vi "Receive Dashboard Packet.vi"(7 "connection ID":refnum<k16>) -> ()   [LabVIEW 2015]
uses:
  Common Code/Dashboard Communication/Dashboard Control Data.ctl
  Common Code/Shooter Presets.ctl
  Common Code/Shot Presets.ctl
  Common Code/Encoder Control.ctl
  Common Code/Drivetrain Settings.ctl
  Common Code/Vision Packet.ctl
  Common Code/Dashboard Drivetrain Command.ctl
  Common Code/Drivetrain Vision.ctl
  Robot Global Data.vi
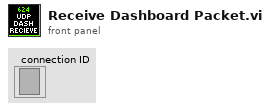
[diagram p1: front panel]
types:
  T1 = typedef "Dashboard Control Data.ctl" = cluster{"Auton Loops":dbl, "Shooter Presets":T2, "Encoder Control":T4, "Steer PID output":cluster{"output high":dbl, "output low":dbl}, " Steer PID gains":cluster{"proportional gain (Kc)":dbl, "integral time (Ti, min)":dbl, "derivative time (Td, min)":dbl}, "Drivetrain Settings":T5, "Vision Packet":T6, "Dashboard Drivetrain Command":T7}
  T2 = typedef "Shooter Presets.ctl" = cluster{"Batter Shot":T3, "Low Bar Curve Shot":T3, "Deep Middle Shot":T3, "Manual Shot":T3}
  T3 = typedef "Shot Presets.ctl" = cluster{"Left Wheel RPM":dbl, "Right Wheel RPM":dbl}
  T4 = typedef "Encoder Control.ctl" = cluster{"Right Tick Constat":dbl, "Left Tick Constant":dbl, "Reset?":bool, "Y Dist":cluster{"PID gains":cluster{"proportional gain (Kc)":dbl, "integral time (Ti, min)":dbl, "derivative time (Td, min)":dbl}}, "Y Stop Thresh":dbl, "Y Stop Speed":dbl}
  T5 = typedef "Drivetrain Settings.ctl" = cluster{"Gyro Tolerance":dbl, "Throttle Ramp (ms)":dbl, "Angular rate compensation":bool, "Throttle to Rate Scale":dbl, "Rate compensation gain":dbl}
  T6 = typedef "Vision Packet.ctl" = cluster{"Distance":dbl, "Center X":dbl, "Center Y":dbl, "Found Target?":bool}
  T7 = typedef "Dashboard Drivetrain Command.ctl" = cluster{"Drivetrain Vision":T8, "Vision Scale Down Speed":dbl, "Vision PID gains":cluster{"proportional gain (Kc)":dbl, "integral time (Ti, min)":dbl, "derivative time (Td, min)":dbl}}
  T8 = typedef "Drivetrain Vision.ctl" = cluster{"High parameters":dbl, "Low parameters":dbl}
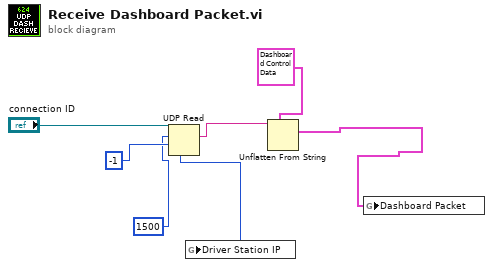
[diagram p0: block diagram]
diagram:
  n1 = UDP Read(connection ID="connection ID", max size (548)=1500, timeout ms (25000)=-1) -> (data out=w4:string, 6:w2:u32)  [unwired: 1 in, 3 out]
  n2 = global write "Robot Global Data.vi" "Driver Station IP"(w2) -> ()
  n3 = Unflatten From String(type=T1 {"Auton Loops"=0.0, "Shooter Presets"={"Batter Shot"={"Left Wheel RPM"=0.0, "Right Wheel RPM"=0.0}, "Low Bar Curve Shot"={"Left Wheel RPM"=0.0, "Right Wheel RPM"=0.0}, "Deep Middle Shot"={"Left Wheel RPM"=0.0, "Right Wheel RPM"=0.0}, "Manual Shot"={"Left Wheel RPM"=0.0, "Right Wheel RPM"=0.0}}, "Encoder Control"={"Right Tick Constat"=0.0, "Left Tick Constant"=0.0, "Reset?"=FALSE, "Y Dist"={"PID gains"={"proportional gain (Kc)"=0.0, "integral time (Ti, min)"=0.0, "derivative time (Td, min)"=0.0}}, "Y Stop Thresh"=0.0, "Y Stop Speed"=0.0}, "Steer PID output"={"output high"=0.0, "output low"=0.0}, " Steer PID gains"={"proportional gain (Kc)"=0.0, "integral time (Ti, min)"=0.0, "derivative time (Td, min)"=0.0}, "Drivetrain Settings"={"Gyro Tolerance"=0.0, "Throttle Ramp (ms)"=0.0, "Angular rate compensation"=FALSE, "Throttle to Rate Scale"=0.0, "Rate compensation gain"=0.0}, "Vision Packet"={"Distance"=0.0, "Center X"=0.0, "Center Y"=0.0, "Found Target?"=FALSE}, "Dashboard Drivetrain Command"={"Drivetrain Vision"={"High parameters"=0.0, "Low parameters"=0.0}, "Vision Scale Down Speed"=0.0, "Vision PID gains"={"proportional gain (Kc)"=1.0, "integral time (Ti, min)"=0.01, "derivative time (Td, min)"=0.0}}} ("Dashboard Control Data"), binary string=w4) -> (value=w1:T1)  [unwired: 3 in, 2 out]
  n4 = global write "Robot Global Data.vi" "Dashboard Packet"(w1) -> ()
